vi "Determine More Warnings.vi"(6 "Max Wind Speed":dbl, 7 "Current Wind Speed":dbl, 9 "Min Temp":dbl, 10 "Max Temp":dbl, 11 "Current Temp":dbl) -> (1 "Warning?":bool, 2 "Warning Text":string)   [LabVIEW 2014]
doc: "This VI is an exercise in the LabVIEW Core I course. In this exercise, you generate appropriate strings for Freeze, Heat Stroke, and High Wind warnings, and combinations of the warnings."
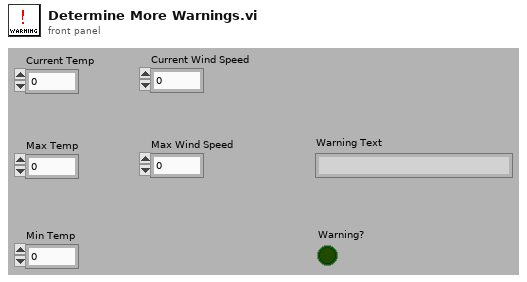
[diagram p1: front panel]
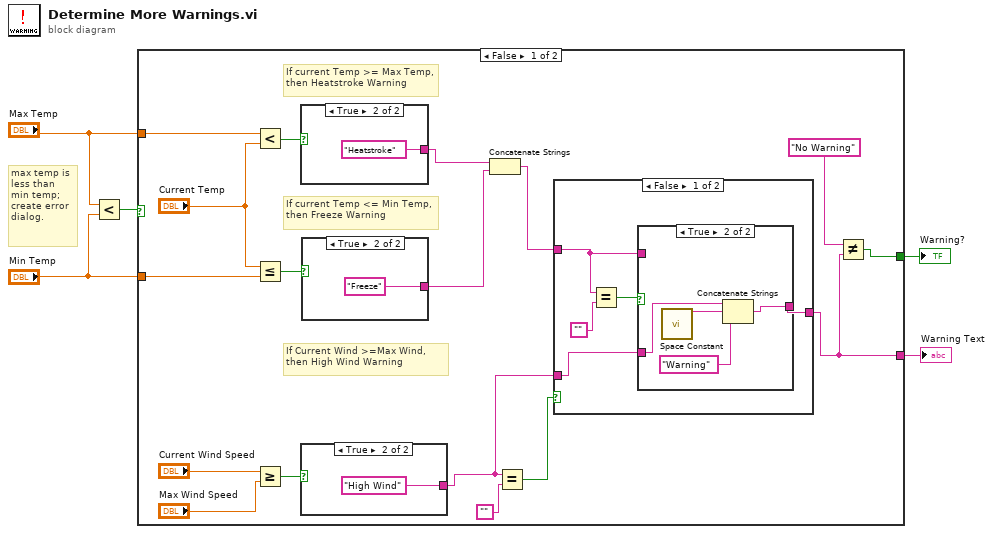
[diagram p0: block diagram]
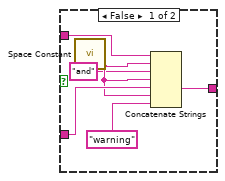
[diagram p2: hidden frame]
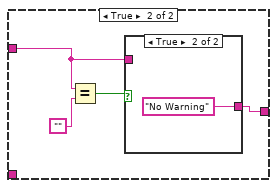
[diagram p3: hidden frame]
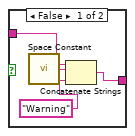
[diagram p4: hidden frame]
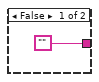
[diagram p5: hidden frame]
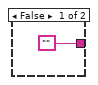
[diagram p6: hidden frame]
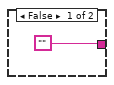
[diagram p7: hidden frame]
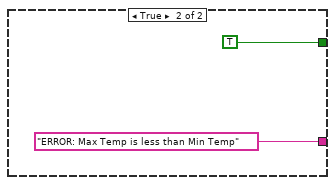
[diagram p8: hidden frame]
diagram:
  # "max temp is less than min temp; create error dialog."
  n1 = Less?(x="Max Temp", y="Min Temp") -> (x < y?=w1:bool)
  n2 = case shown="False" w1 {
    tunnel: [w8 TRUE] -> w5
    tunnel: [w7 "ERROR: Max Temp is less than Min Temp"] -> w4
    tunnel: "Max Temp" -> [w16 _]
    tunnel: "Min Temp" -> [w15 _]
    frame False {
      # "If Current Wind >=Max Wind, then High Wind Warning"
      # "If current Temp <= Min Temp, then Freeze Warning"
      # "If current Temp >= Max Temp, then Heatstroke Warning"
      n3 = Less?(x=w16, y="Current Temp") -> (x < y?=w20:bool)
      n4 = Less Or Equal?(x="Current Temp", y=w15) -> (x <= y?=w22:bool)
      n5 = Greater Or Equal?(x="Current Wind Speed", y="Max Wind Speed") -> (x >= y?=w17:bool)
      n6 = case shown="True" w20 {
        tunnel: ["" "Heatstroke"] -> w14
        frame False {
        }
        frame True {
        }
      }
      n7 = case shown="True" w17 {
        tunnel: ["" "High Wind"] -> w10
        frame False {
        }
        frame True {
        }
      }
      n8 = case shown="True" w22 {
        tunnel: ["" "Freeze"] -> w13
        frame False {
        }
        frame True {
        }
      }
      n9 = Concatenate Strings(w14, w13) -> (w11:string)
      n10 = Equal?(x=w10, y="") -> (x = y?=w9:bool)
      n11 = case shown="False" w9 {
        tunnel: w11 -> [w25 w39]
        tunnel: w10 -> [w23 _]
        tunnel: [w24 w38] -> w7
        frame False {
          n12 = Equal?(x=w25, y="") -> (x = y?=w26:bool)
          n13 = case shown="True" w26 {
            tunnel: w25 -> [w32 _]
            tunnel: [w33 w37] -> w24
            tunnel: w23 -> [w31 w36]
            frame False {
              n14 = call <vilib>:"Space Constant.vi"() -> ("String"=w30:string)
              n15 = Concatenate Strings(w32, w30, "and", w30, w31, w30, "warning") -> (w33:string)
            }
            frame True {
              n16 = call <vilib>:"Space Constant.vi"() -> ("String"=w35:string)
              n17 = Concatenate Strings(w36, w35, "Warning") -> (w37:string)
            }
          }
        }
        frame True {
          n18 = Equal?(x=w39, y="") -> (x = y?=w40:bool)
          n19 = case shown="True" w40 {
            tunnel: w39 -> [w42 _]
            tunnel: [w45 "No Warning"] -> w38
            frame False {
              n20 = call <vilib>:"Space Constant.vi"() -> ("String"=w43:string)
              n21 = Concatenate Strings(w42, w43, "Warning") -> (w45:string)
            }
            frame True {
            }
          }
        }
      }
      n22 = Not Equal?(x="No Warning", y=w7) -> (x != y?=w8:bool)
    }
    frame True {
    }
  }
  "Warning Text" <- w4
  "Warning?" <- w5
